vi "Connection Ref.vi"(11 "TCP Comm":T1) -> (3 "TCP":refnum<k5>)   [LabVIEW 2020, in "TCP Comms.lvlib"]
uses:
  TCP Comms.lvlib
  TCP Comm.ctl
  Ref Data.ctl
  State.ctl
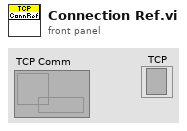
[diagram p1: front panel]
types:
  T1 = typedef "TCP Comms.lvlib/TCP Comm.ctl" = refnum<data-value>
  T2 = typedef "TCP Comms.lvlib/Ref Data.ctl" = cluster{"TCP":refnum<k5>, "State":T3, "Server":bool, "Host":string, "Port":u16, "Listener":refnum<k5>, "Start":bool, "Disconnect":bool, "TCP Valid":bool, "TLS Enabled":bool, "Immutable TLS":refnum<k36>, "Certificate DN":string}
  T3 = typedef "TCP Comms.lvlib/State.ctl" = enum16{"Idle", "Starting", "Connecting", "Connected", "Disconnecting", "Stopped"}
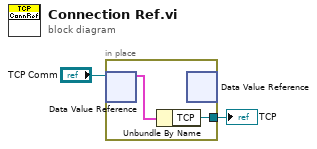
[diagram p0: block diagram]
diagram:
  n1 = in-place {
    in-place-border: [w3] -> w1
    n2 = in-place-dvr #1("TCP Comm") -> (w4:T2)  [unwired: 1 out]
    n3 = Unbundle By Name(w4) -> ("TCP"=w3:refnum<k5>)
    n4 = in-place-dvr #1() -> ()  [unwired: 1 in, 2 out]
  }
  "TCP" <- w1
